vi "Setup For StdOut.vi"(4 "error in (no error)":errorcluster) -> (0 "error out":errorcluster)   [LabVIEW 2015, in "StdOut Operations.lvlib"]
uses:
  StdOut Operations.lvlib
  kernel32.dll
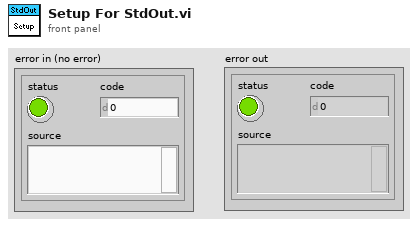
[diagram p1: front panel]
types:
  T1 = enum16{"Duplication Failed", "Duplication Succeeded"}
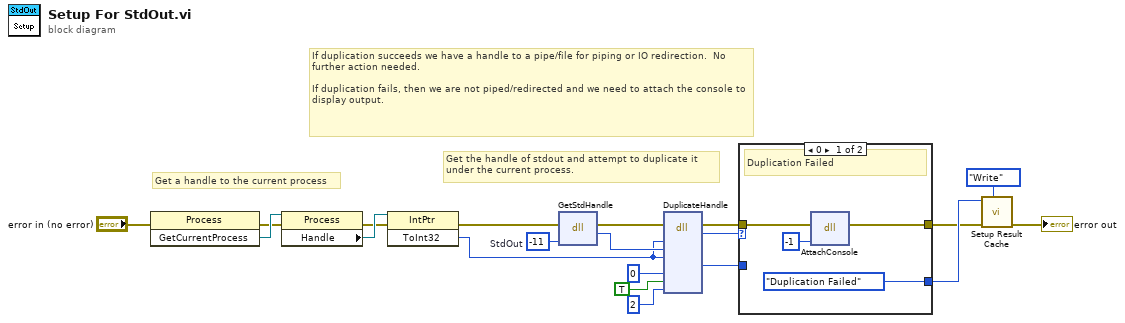
[diagram p0: block diagram]
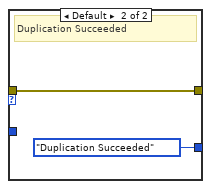
[diagram p2: hidden frame]
diagram:
  w13 = -11  # StdOut
  # "If duplication succeeds we have a handle to a pipe/file for piping or IO redirection.  No further action needed.\n\nIf duplication fails, then we are not piped/redirected and we need to attach the console to display output."
  # "Get the handle of stdout and attempt to duplicate it\nunder the current process."
  # "Get a handle to the current process"
  n1 = invoke class="Process" method="GetCurrentProcess"(error in="error in (no error)") -> (error out=w6:errorcluster, "GetCurrentProcess"=w15:refnum<k24>)  [unwired: 2 in, 1 out]
  n2 = property class="Process"(reference=w15, error in=w6) -> (error out=w7:errorcluster, "Handle"=w16:refnum<k24>)  [unwired: 1 out]
  n3 = invoke class="IntPtr" method="ToInt32"(reference=w16, error in=w7) -> (error out=w12:errorcluster, "ToInt32"=w5:i32)  [unwired: 1 in, 1 out]
  n4 = dll-call lib="kernel32.dll" fn="GetStdHandle"(error in=w12, "nStdHandle"=w13) -> (error out=w17:errorcluster, "return type"=w14:i32)  [unwired: 3 in, 1 out]
  n5 = dll-call lib="kernel32.dll" fn="DuplicateHandle"(error in=w17, "hSourceProcess"=w5, "hSourceHandle"=w14, "hTargetProcess"=w5, "dwDesirecAccess"=u16 0, "bInheritHandle"=TRUE, "dwOptions"=u16 2) -> (error out=w8:errorcluster, "return type"=w18:u8, "lpTargetHandle"=w19:i32)  [unwired: 9 in, 1 out]
  n6 = case shown="0" w18 {
    tunnel: w8 -> [w24 w26]
    tunnel: [w23 w26] -> w3
    tunnel: w19 -> [_ _]
    tunnel: [T1."Duplication Failed" ("Result") T1."Duplication Succeeded" ("Result")] -> w4
    frame 0 {
      # "Duplication Failed"
      n7 = dll-call lib="kernel32.dll" fn="AttachConsole"(error in=w24, "arg1"=-1) -> (error out=w23:errorcluster)  [unwired: 4 in, 1 out]
    }
    frame Default {
      # "Duplication Succeeded"
    }
  }
  n8 = call "Setup Result Cache.vi"("Operation"=enum16{"Read", "Write"}."Write", "error in (no error)"=w3, "Result"=w4) -> ("error out"=→"error out":errorcluster)  [unwired: 4 in, 1 out]
